vi "NPL Joerger Dust Ablation.vi"() -> ()   [LabVIEW 2013]
uses:
  <vilib>/Utility/file.llb/Write To Spreadsheet File (DBL).vi
panel:
  out "Event Num":i32
  out "Waveforms":ext[][](graph)
  out "Waveform 17-32":ext[][](graph)
  out "State":i32
  in  "Save Files":bool
  out "Waveform output":ext[][](array[numeric])
  out "8bit integer 3":i8 format="%08b"
  out "8bit integer 2":i8 format="%08b"
  out "8bit integer":i8 format="%08b"
  out "dt":dbl
  in  "Change folder":bool
  out "Waveform Folder":path
  in  "Manual Arm":bool
  out "Waveform 1-16":ext[][](graph)
  out "# Channels Plotted":i32
  in  "How Many Cards?":u16(ring) items=["2", "3"]
  out "Electrons Min Signal":cluster{i32[], "Ions Max Value":ext[]}(graph)
  out "Ions Max Signal":cluster{i32[], "Ions Max Value":ext[]}(graph)
  out "Sec. Since Last Read":dbl
  in  "stop":bool
  in  "Arm":bool
  in  "Number of Channels":u8=16
  in  "# Samples":u32=2000 min=1 max=262143 step=1
  out "Length of Sample":dbl caption="s" format="%^#_3g"
  in  "Acquisition Rate 2":u16(ring)=2 items=["40 MHz", "20 MHz", "10 MHz", "5 MHz", "2.5 MHz", "1 MHz", "100 kHz", "10 kHz"]
  # "0"
  # "1"
  # "Sampling Controls"
  # "Sampling Info"
  # "Triggering Setup"
  # "2"
  # "3"
  # "4"
  # "5"
  # "6"
  # "7"
  # "8"
  # "9"
  # "10"
  # "11"
  # "This resets the\nwaveform count \nto zero when saving\nwaveforms"
  # "12"
  # "13"
  # "14"
  # "15"
  # "0"
  # "1"
  # "2"
  # "3"
  # "4"
  # "5"
  # "6"
  # "7"
  # "8"
  # "9"
  # "10"
  # "11"
  # "12"
  # "13"
  # "14"
  # "15"
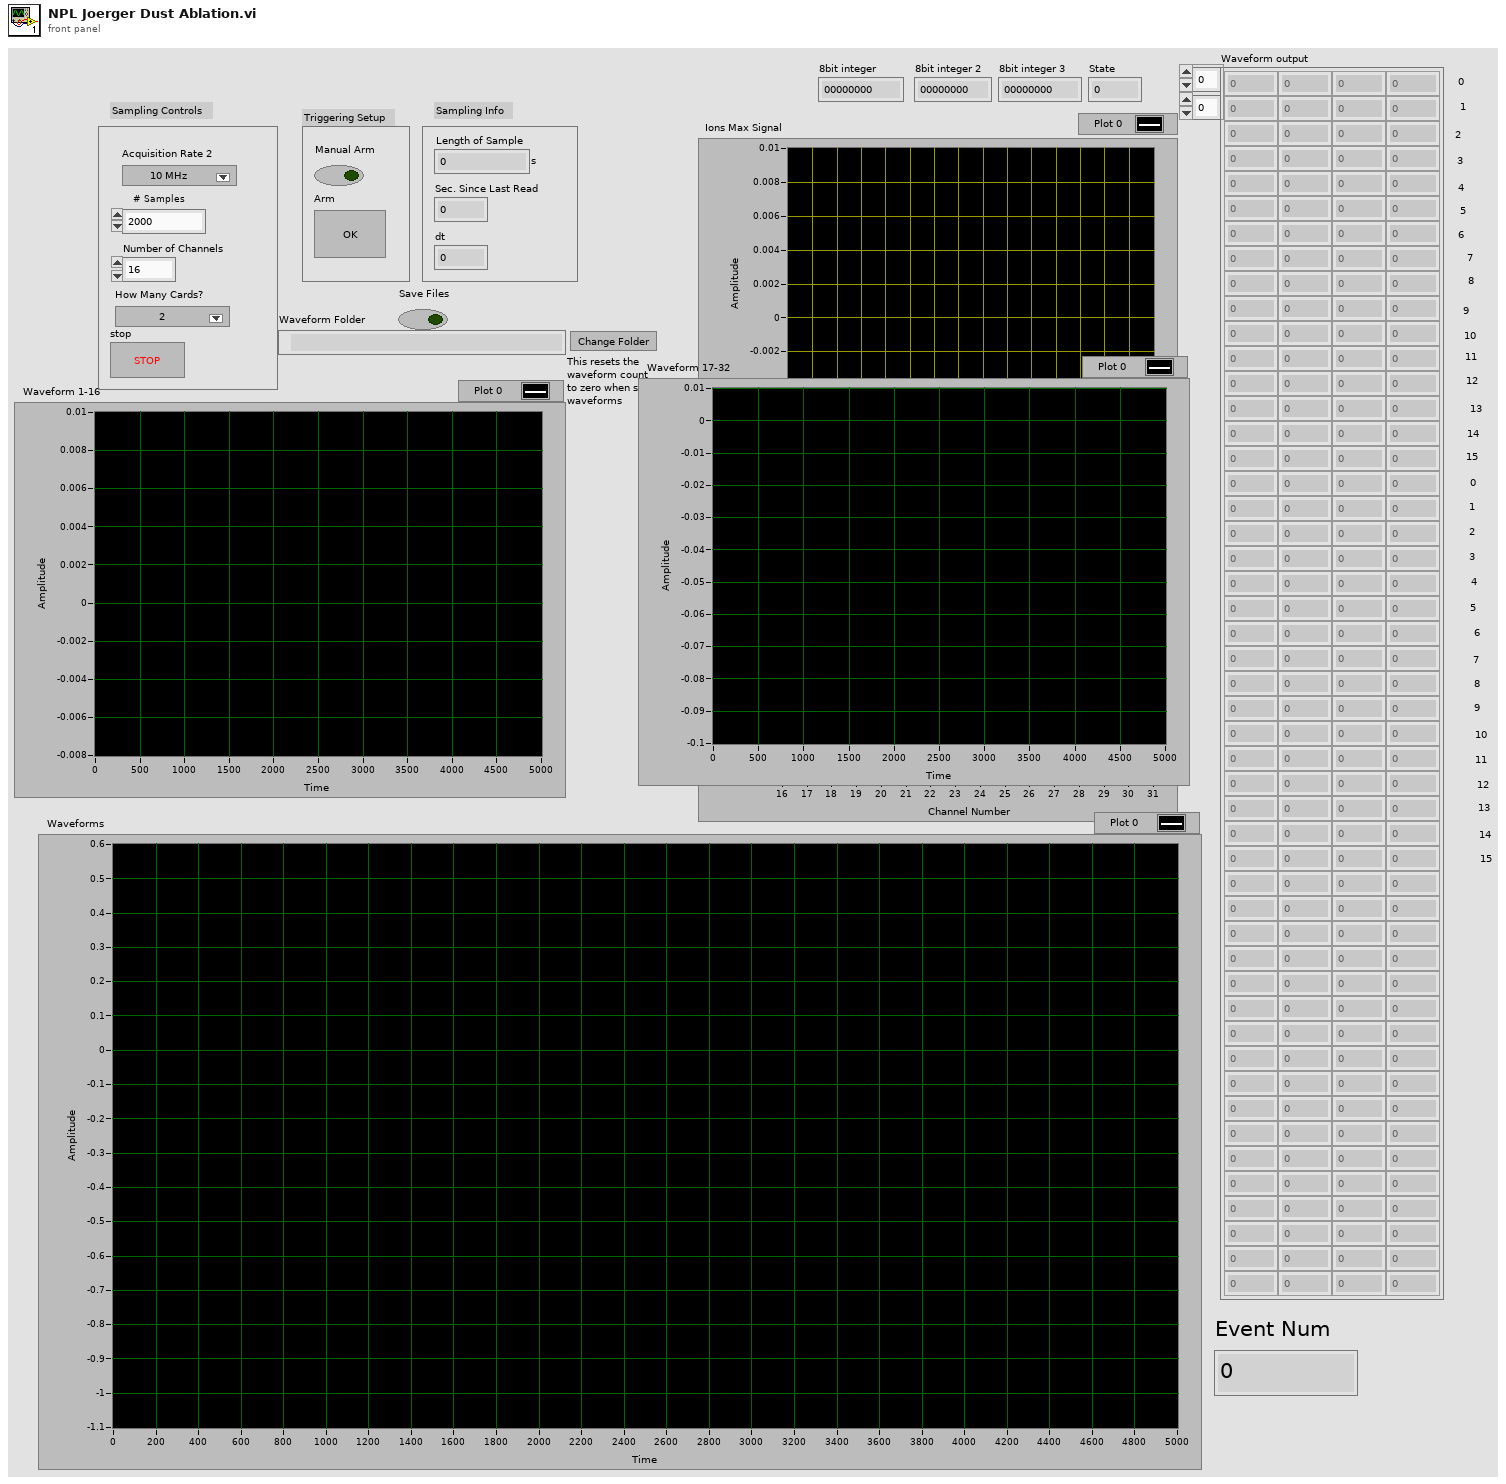
[diagram p1: front panel]
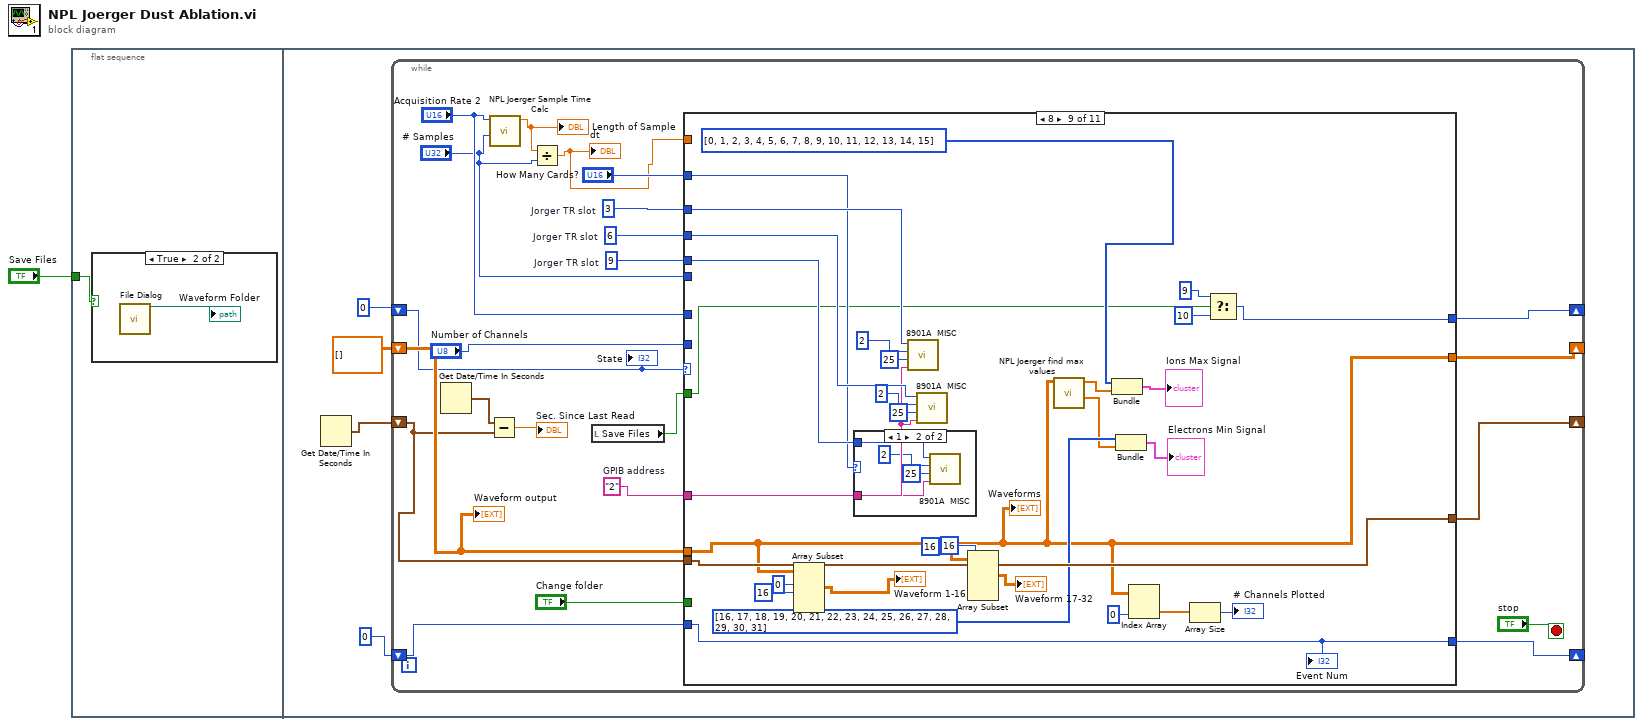
[diagram p0: block diagram]
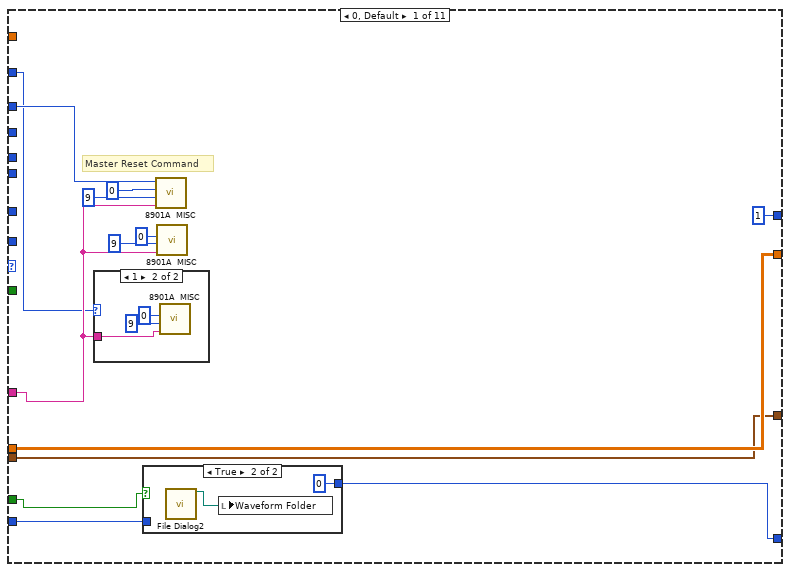
[diagram p3: hidden frame]
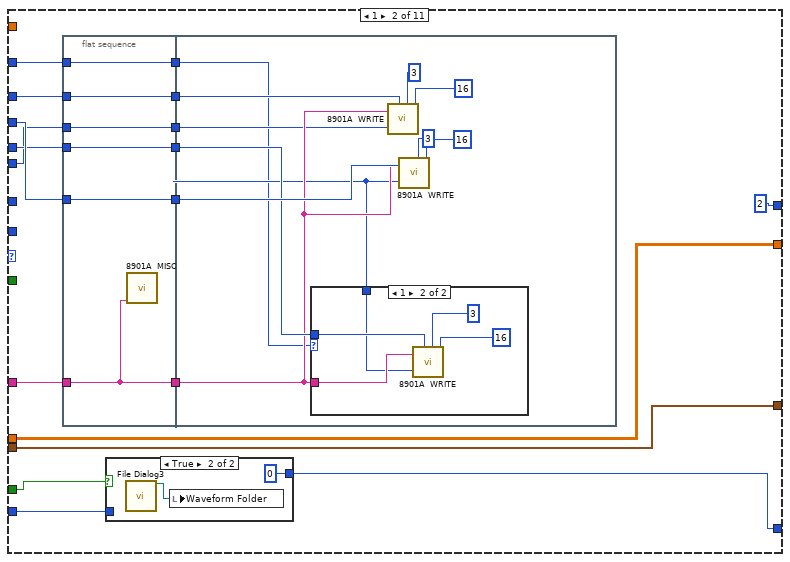
[diagram p6: hidden frame]
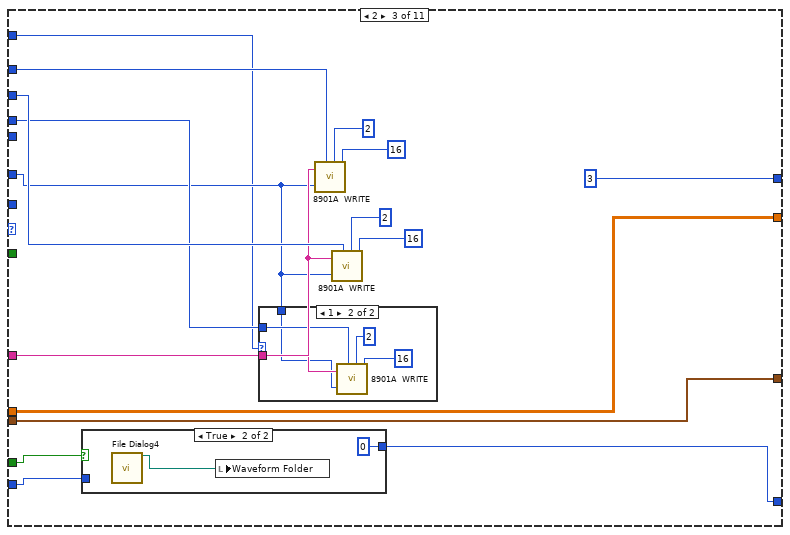
[diagram p9: hidden frame]
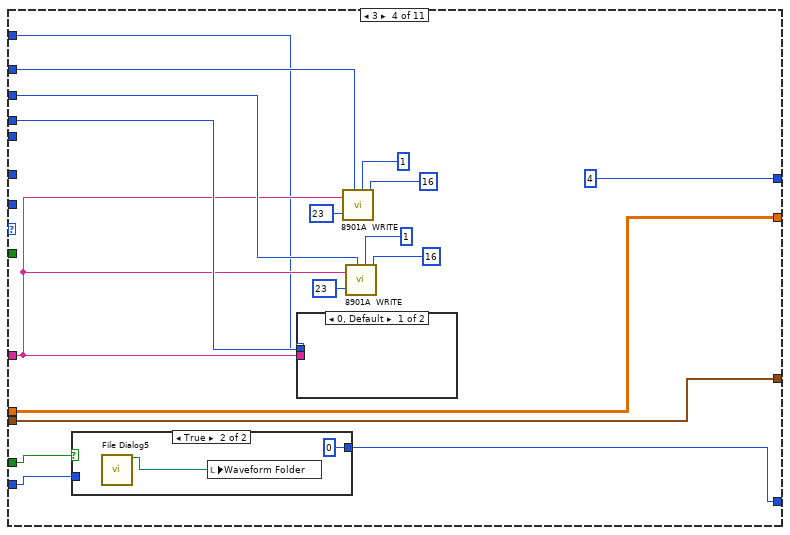
[diagram p12: hidden frame]
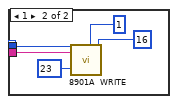
[diagram p14: hidden frame]
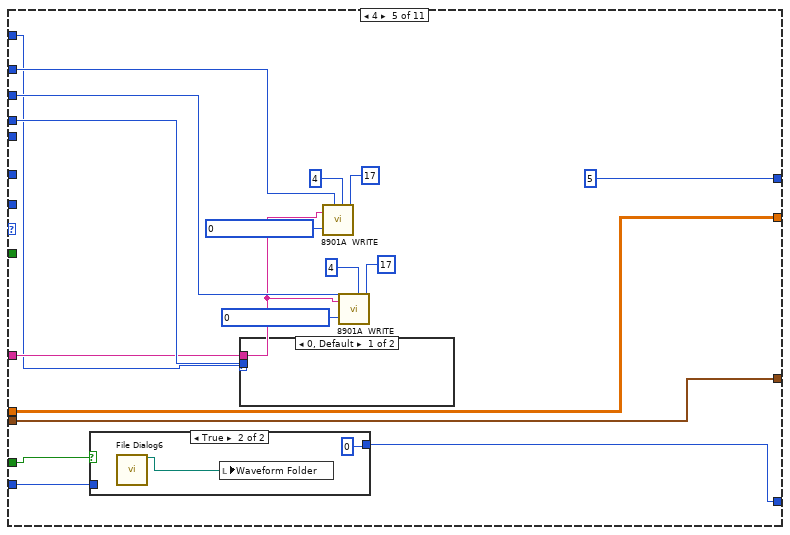
[diagram p15: hidden frame]
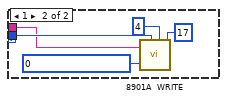
[diagram p17: hidden frame]
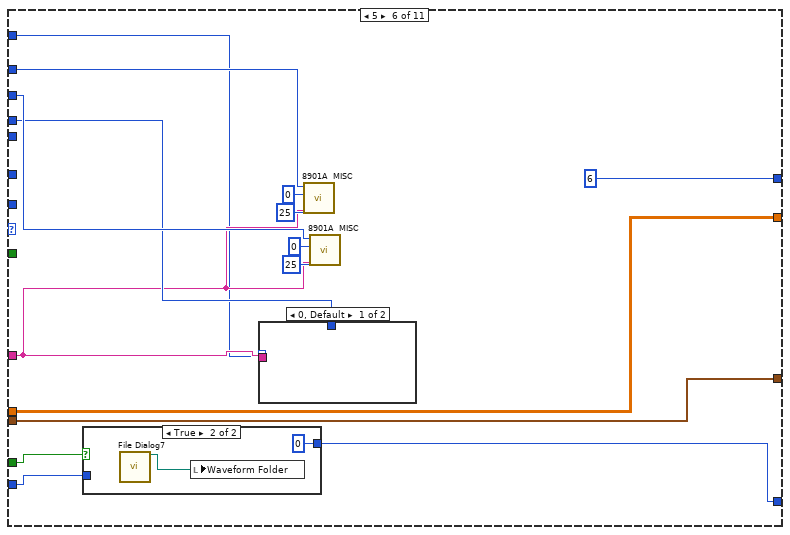
[diagram p18: hidden frame]
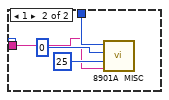
[diagram p20: hidden frame]
diagram:
  n1 = flat-sequence {
    tunnel: "Save Files" -> [w2]
    frame #0 {
      n2 = case shown="True" w2 {
        frame False {
        }
        frame True {
          n3 = call "File Dialog"() -> ("selected path"=→"Waveform Folder":path)  [unwired: 12 in, 3 out]
        }
      }
    }
    frame #1 {
      n4 = Get Date/Time In Seconds() -> (seconds since 1Jan1904=w5:timestamp)
      n5 = while {
        shift-right: [w28] -> _
        shift-left: 0 -> [w23]
        shift-right: [w25] -> _
        shift-left: ext[][] [] ("output") -> [w24]
        shift-right: [w22] -> _
        shift-left: w5 -> [w20]
        shift-right: [w12] -> _
        shift-left: 0 -> [w13]
        stop <- "stop" stop-if-true
        w17 = u8 9  # Jorger TR slot
        w18 = u8 6  # Jorger TR slot
        w30 = u8 3  # Jorger TR slot
        w29 = "2"  # GPIB address
        n6 = Get Date/Time In Seconds() -> (seconds since 1Jan1904=w21:timestamp)
        n7 = Subtract(x=w21, y=w20) -> (x-y=→"Sec. Since Last Read":dbl)
        n8 = call "NPL Joerger Sample Time Calc.vi"("# Samples"="# Samples", "Acquisition Rate"="Acquisition Rate 2") -> ("Sample Time"=w11:dbl)  [unwired: 9 in]
        "Length of Sample" <- w11
        n9 = Divide(x=w11, y="# Samples") -> (x/y=w9:dbl)
        "dt" <- w9
        n10 = local read "Save Files"() -> (w8:bool)
        n11 = case shown="8" w23 {
          tunnel: w30 -> [w37 w67 w107 w132 w157 w180 w226 w262 w355 _ _]
          tunnel: w29 -> [w38 w61 w97 w120 w145 w170 w197 w263 w347 _ _]
          tunnel: [1 ("f") 2 3 4 5 6 w199 8 ("f") w332 10 ("f") w387] -> w28
          tunnel: "# Samples" -> [_ w60 _ _ _ _ _ w259 _ _ _]
          tunnel: "Acquisition Rate 2" -> [_ _ w96 _ _ _ _ _ _ _ _]
          tunnel: "Number of Channels" -> [_ _ _ _ _ _ _ w260 _ _ _]
          tunnel: [w43 w65 w103 w127 w152 w176 w212 w248 w325 w378 w386] -> w25
          tunnel: w24 -> [w43 w65 w103 w127 w152 w176 w212 _ w325 w378 w386]
          tunnel: w20 -> [w42 w64 w102 w126 w151 w175 w211 _ w352 w366 w389]
          tunnel: [w42 w64 w102 w126 w151 w175 w211 w258 w352 w366 w389] -> w22
          tunnel: w18 -> [_ w63 w99 w122 w147 w172 w208 w256 w349 _ _]
          tunnel: w17 -> [_ w62 w98 w121 w146 w171 w198 w255 w348 _ _]
          tunnel: "How Many Cards?" -> [w31 w59 w95 w119 w144 w169 w191 w247 w340 _ _]
          tunnel: "Change folder" -> [w41 w58 w94 w118 w143 w168 w190 _ _ _ _]
          tunnel: w13 -> [w39 w56 w92 w116 w141 w166 w188 w246 w336 w369 w385]
          tunnel: [w40 w57 w93 w117 w142 w167 w189 w245 w336 w369 w385] -> w12
          tunnel: w9 -> [_ _ _ _ _ _ _ _ _ w368 _]
          tunnel: w8 -> [_ _ _ _ _ _ _ _ w335 _ _]
          frame 0, Default {
            # "Master Reset Command"
            n12 = case shown="1" w31 {
              tunnel: w38 -> [_ w46]
              frame 0, Default {
              }
              frame 1 {
                n13 = call <instrlib>:"8901A  MISC.vi"("GPIB address"=w46, "f"=u8 9, "a"=u8 0) -> ()  [unwired: 1 in]
              }
            }
            n14 = case shown="True" w41 {
              tunnel: [w47 0] -> w40
              tunnel: w39 -> [w47 _]
              frame False {
              }
              frame True {
                n15 = call "File Dialog2"() -> ("selected path"=w49:path)  [unwired: 12 in, 3 out]
                n16 = local write "Waveform Folder"(w49) -> ()
              }
            }
            n17 = call <instrlib>:"8901A  MISC.vi"("GPIB address"=w38, "f"=u8 9, "a"=u8 0, "n"=w37) -> ()
            n18 = call <instrlib>:"8901A  MISC.vi"("GPIB address"=w38, "f"=u8 9, "a"=u8 0) -> ()  [unwired: 1 in]
          }
          frame 1 {
            n19 = flat-sequence {
              tunnel: w59 -> [w69]
              tunnel: w60 -> [w70]
              tunnel: w61 -> [w68]
              tunnel: w62 -> [w71]
              tunnel: w63 -> [w72]
              tunnel: w67 -> [w73]
              tunnel: [w73] -> w55
              tunnel: [w72] -> w54
              tunnel: [w71] -> w53
              tunnel: [w68] -> w52
              tunnel: [w70] -> w51
              tunnel: [w69] -> w50
              tunnel: w55 -> [w83]
              tunnel: w54 -> [w78]
              tunnel: w53 -> [w77]
              tunnel: w52 -> [w76]
              tunnel: w51 -> [w75]
              tunnel: w50 -> [w74]
              frame #0 {
                n20 = call <instrlib>:"8901A  MISC.vi"("GPIB address"=w68) -> ()  [unwired: 3 in]
              }
              frame #1 {
                n21 = case shown="1" w74 {
                  tunnel: w77 -> [_ w86]
                  tunnel: w76 -> [_ w85]
                  tunnel: w75 -> [_ w84]
                  frame 0, Default {
                  }
                  frame 1 {
                    n22 = call <instrlib>:"8901A  WRITE.vi"("data"=w84, "GPIB address"=w85, "n"=w86, "a"=u8 3, "f"=u8 16) -> ()  [unwired: 1 in]
                  }
                }
                n23 = call <instrlib>:"8901A  WRITE.vi"("data"=w75, "GPIB address"=w76, "n"=w83, "a"=u8 3, "f"=u8 16) -> ()  [unwired: 1 in]
                n24 = call <instrlib>:"8901A  WRITE.vi"("data"=w75, "GPIB address"=w76, "n"=w78, "a"=u8 3, "f"=u8 16) -> ()  [unwired: 1 in]
              }
            }
            n25 = case shown="True" w58 {
              tunnel: [w89 0] -> w57
              tunnel: w56 -> [w89 _]
              frame False {
              }
              frame True {
                n26 = call "File Dialog3"() -> ("selected path"=w91:path)  [unwired: 12 in, 3 out]
                n27 = local write "Waveform Folder"(w91) -> ()
              }
            }
          }
          frame 2 {
            n28 = case shown="True" w94 {
              tunnel: [w108 0] -> w93
              tunnel: w92 -> [w108 _]
              frame False {
              }
              frame True {
                n29 = call "File Dialog4"() -> ("selected path"=w110:path)  [unwired: 12 in, 3 out]
                n30 = local write "Waveform Folder"(w110) -> ()
              }
            }
            n31 = case shown="1" w95 {
              tunnel: w98 -> [_ w113]
              tunnel: w97 -> [_ w112]
              tunnel: w96 -> [_ w111]
              frame 0, Default {
              }
              frame 1 {
                n32 = call <instrlib>:"8901A  WRITE.vi"("data"=w111, "GPIB address"=w112, "n"=w113, "a"=u8 2, "f"=u8 16) -> ()  [unwired: 1 in]
              }
            }
            n33 = call <instrlib>:"8901A  WRITE.vi"("data"=w96, "GPIB address"=w97, "n"=w107, "a"=u8 2, "f"=u8 16) -> ()  [unwired: 1 in]
            n34 = call <instrlib>:"8901A  WRITE.vi"("data"=w96, "GPIB address"=w97, "n"=w99, "a"=u8 2, "f"=u8 16) -> ()  [unwired: 1 in]
          }
          frame 3 {
            n35 = case shown="True" w118 {
              tunnel: [w133 0] -> w117
              tunnel: w116 -> [w133 _]
              frame False {
              }
              frame True {
                n36 = call "File Dialog5"() -> ("selected path"=w135:path)  [unwired: 12 in, 3 out]
                n37 = local write "Waveform Folder"(w135) -> ()
              }
            }
            n38 = case shown="0, Default" w119 {
              tunnel: w121 -> [_ w137]
              tunnel: w120 -> [_ w136]
              frame 0, Default {
              }
              frame 1 {
                n39 = call <instrlib>:"8901A  WRITE.vi"("data"=23, "GPIB address"=w136, "n"=w137, "a"=u8 1, "f"=u8 16) -> ()  [unwired: 1 in]
              }
            }
            n40 = call <instrlib>:"8901A  WRITE.vi"("data"=23, "GPIB address"=w120, "n"=w132, "a"=u8 1, "f"=u8 16) -> ()  [unwired: 1 in]
            n41 = call <instrlib>:"8901A  WRITE.vi"("data"=23, "GPIB address"=w120, "n"=w122, "a"=u8 1, "f"=u8 16) -> ()  [unwired: 1 in]
          }
          frame 4 {
            n42 = case shown="True" w143 {
              tunnel: [w158 0] -> w142
              tunnel: w141 -> [w158 _]
              frame False {
              }
              frame True {
                n43 = call "File Dialog6"() -> ("selected path"=w160:path)  [unwired: 12 in, 3 out]
                n44 = local write "Waveform Folder"(w160) -> ()
              }
            }
            n45 = case shown="0, Default" w144 {
              tunnel: w146 -> [_ w162]
              tunnel: w145 -> [_ w161]
              frame 0, Default {
              }
              frame 1 {
                n46 = call <instrlib>:"8901A  WRITE.vi"("data"=0, "GPIB address"=w161, "n"=w162, "a"=u8 4, "f"=u8 17) -> ()  [unwired: 1 in]
              }
            }
            n47 = call <instrlib>:"8901A  WRITE.vi"("data"=0, "GPIB address"=w145, "n"=w157, "a"=u8 4, "f"=u8 17) -> ()  [unwired: 1 in]
            n48 = call <instrlib>:"8901A  WRITE.vi"("data"=0, "GPIB address"=w145, "n"=w147, "a"=u8 4, "f"=u8 17) -> ()  [unwired: 1 in]
          }
          frame 5 {
            n49 = case shown="True" w168 {
              tunnel: [w181 0] -> w167
              tunnel: w166 -> [w181 _]
              frame False {
              }
              frame True {
                n50 = call "File Dialog7"() -> ("selected path"=w183:path)  [unwired: 12 in, 3 out]
                n51 = local write "Waveform Folder"(w183) -> ()
              }
            }
            n52 = case shown="0, Default" w169 {
              tunnel: w171 -> [_ w185]
              tunnel: w170 -> [_ w184]
              frame 0, Default {
              }
              frame 1 {
                n53 = call <instrlib>:"8901A  MISC.vi"("GPIB address"=w184, "f"=u8 25, "a"=u8 0, "n"=w185) -> ()
              }
            }
            n54 = call <instrlib>:"8901A  MISC.vi"("GPIB address"=w170, "f"=u8 25, "a"=u8 0, "n"=w180) -> ()
            n55 = call <instrlib>:"8901A  MISC.vi"("GPIB address"=w170, "f"=u8 25, "a"=u8 0, "n"=w172) -> ()
          }
          frame 6 {
            # "Check status register to see that\nmodule is neither armed nor active\n(bits R1 & R2 = 0)."
            n56 = case shown="True" w190 {
              tunnel: [w227 0] -> w189
              tunnel: w188 -> [w227 _]
              frame False {
              }
              frame True {
                n57 = call "File Dialog8"() -> ("selected path"=w229:path)  [unwired: 12 in, 3 out]
                n58 = local write "Waveform Folder"(w229) -> ()
              }
            }
            n59 = case shown="1" w191 {
              tunnel: w198 -> [_ w242]
              tunnel: w197 -> [_ w241]
              tunnel: [FALSE w231] -> w193
              frame 0, Default {
              }
              frame 1 {
                n60 = call <instrlib>:"8901A READ 8.vi"("GPIB address"=w241, "n"=w242, "a"=u8 0, "f"=u8 1) -> ("output"=w232:ext)  [unwired: 3 in]
                n61 = To Byte Integer(number=w232) -> (8bit integer=w240:i8)
                "8bit integer 3" <- w240
                n62 = And(x=w240, y=i8 3) -> (x .and. y?=w238:i8)
                n63 = Number To Boolean Array(number=w238) -> (Boolean array=w236:bool[])
                n64 = Index Array(array=w236, index=0) -> (element=w233:bool)
                n65 = Index Array(array=w236, index=1) -> (element=w234:bool)
                n66 = Or(x=w233, y=w234) -> (x .or. y?=w231:bool)
              }
            }
            n67 = call <instrlib>:"8901A READ 8.vi"("GPIB address"=w197, "n"=w226, "a"=u8 0, "f"=u8 1) -> ("output"=w223:ext)  [unwired: 3 in]
            n68 = call <instrlib>:"8901A READ 8.vi"("GPIB address"=w197, "n"=w208, "a"=u8 0, "f"=u8 1) -> ("output"=w196:ext)  [unwired: 3 in]
            n69 = To Byte Integer(number=w223) -> (8bit integer=w222:i8)
            "8bit integer" <- w222
            n70 = To Byte Integer(number=w196) -> (8bit integer=w200:i8)
            "8bit integer 2" <- w200
            n71 = And(x=w222, y=i8 3) -> (x .and. y?=w220:i8)
            n72 = And(x=w200, y=i8 3) -> (x .and. y?=w202:i8)
            n73 = Number To Boolean Array(number=w220) -> (Boolean array=w218:bool[])
            n74 = Number To Boolean Array(number=w202) -> (Boolean array=w204:bool[])
            n75 = Index Array(array=w218, index=0) -> (element=w215:bool)
            n76 = Index Array(array=w218, index=1) -> (element=w216:bool)
            n77 = Index Array(array=w204, index=0) -> (element=w207:bool)
            n78 = Index Array(array=w204, index=1) -> (element=w206:bool)
            n79 = Or(x=w215, y=w216) -> (x .or. y?=w195:bool)
            n80 = Or(x=w207, y=w206) -> (x .or. y?=w194:bool)
            n81 = Compound Arithmetic op=OR(w195, w194, w193) -> (w192:bool)
            n82 = Select(t=6, s=w192, f=7) -> (s? t:f=w199:i32)
          }
          frame 7 {
            # "Increment\nWaveform #"
            # "0...15 card 1\n16...31 card 2\n32...47 card 3"
            # "Read out the data from the number of channels\nspecified."
            n83 = Increment(x=w246) -> (x+1=w245:i32)
            n84 = for {
              N: w260 -> [_]
              tunnel: w263 -> [w273]
              tunnel: w262 -> [w283]
              tunnel: w259 -> [w271]
              tunnel: [w280] -> w257 mode=indexing
              tunnel: w256 -> [w277]
              tunnel: [w276] -> w254 mode=indexing
              tunnel: [w275] -> w253 mode=indexing
              tunnel: w255 -> [w274]
              tunnel: w247 -> [w270]
              i -> [w272]
              n85 = case shown="1" w270 {
                tunnel: [ext[] [] ("output") w289] -> w275
                tunnel: w274 -> [_ w288]
                tunnel: w273 -> [_ w287]
                tunnel: w272 -> [_ w286]
                tunnel: w271 -> [_ w285]
                frame 0, Default {
                }
                frame 1 {
                  n86 = flat-sequence {
                    tunnel: w287 -> [w293]
                    tunnel: w288 -> [w292]
                    tunnel: [w293] -> w291
                    tunnel: [w292] -> w290
                    tunnel: w291 -> [w302]
                    tunnel: w290 -> [w301]
                    tunnel: w286 -> [w299]
                    tunnel: [w297] -> _
                    tunnel: [w298] -> w289
                    tunnel: w285 -> [w297]
                    frame #0 {
                      n87 = call <instrlib>:"8901A  WRITE.vi"("data"=0, "GPIB address"=w293, "n"=w292, "a"=u8 1, "f"=u8 17) -> ()  [unwired: 1 in]
                    }
                    frame #1 {
                      n88 = call <instrlib>:"8901A BLOCK READ 24.vi"("f"=u8 2, "a"=w299, "n"=w301, "GPIB address"=w302, "# points to read"=w297) -> ("output"=w298:ext[])  [unwired: 4 in]
                    }
                  }
                }
              }
              n89 = flat-sequence {
                tunnel: w273 -> [w315]
                tunnel: w283 -> [w314]
                tunnel: [w315] -> w282
                tunnel: [w314] -> w281
                tunnel: w282 -> [w324]
                tunnel: w281 -> [w323]
                tunnel: w272 -> [w321]
                tunnel: w271 -> [w320]
                tunnel: [w319] -> w280
                frame #0 {
                  n90 = call <instrlib>:"8901A  WRITE.vi"("data"=0, "GPIB address"=w315, "n"=w314, "a"=u8 1, "f"=u8 17) -> ()  [unwired: 1 in]
                }
                frame #1 {
                  n91 = call <instrlib>:"8901A BLOCK READ 24.vi"("f"=u8 2, "a"=w321, "n"=w323, "GPIB address"=w324, "# points to read"=w320) -> ("output"=w319:ext[])  [unwired: 4 in]
                }
              }
              n92 = flat-sequence {
                tunnel: w273 -> [w304]
                tunnel: w277 -> [w303]
                tunnel: [w304] -> w279
                tunnel: [w303] -> w278
                tunnel: w279 -> [w313]
                tunnel: w278 -> [w312]
                tunnel: w272 -> [w310]
                tunnel: w271 -> [w309]
                tunnel: [w308] -> w276
                frame #0 {
                  n93 = call <instrlib>:"8901A  WRITE.vi"("data"=0, "GPIB address"=w304, "n"=w303, "a"=u8 1, "f"=u8 17) -> ()  [unwired: 1 in]
                }
                frame #1 {
                  n94 = call <instrlib>:"8901A BLOCK READ 24.vi"("f"=u8 2, "a"=w310, "n"=w312, "GPIB address"=w313, "# points to read"=w309) -> ("output"=w308:ext[])  [unwired: 4 in]
                }
              }
            }
            n95 = call "NPL Joerger ADC Convert.vi"("Input"=w257) -> ("Output"=w252:ext[][])  [unwired: 10 in]
            n96 = call "NPL Joerger ADC Convert.vi"("Input"=w254) -> ("Output"=w250:ext[][])  [unwired: 10 in]
            n97 = Insert Into Array(array=w252, index (row)=16, new element=w250) -> (w249:ext[][])  [unwired: 1 in]
            n98 = case shown="1" w247 {
              tunnel: w253 -> [_ w269]
              tunnel: w249 -> [w264 w268]
              tunnel: [w264 w265] -> w248
              frame 0, Default {
              }
              frame 1 {
                n99 = call "NPL Joerger ADC Convert.vi"("Input"=w269) -> ("Output"=w266:ext[][])  [unwired: 10 in]
                n100 = Insert Into Array(array=w268, index (row)=32, new element=w266) -> (w265:ext[][])  [unwired: 1 in]
              }
            }
            n101 = Get Date/Time In Seconds() -> (seconds since 1Jan1904=w258:timestamp)
          }
          frame 8 {
            n102 = Array Subset(array=w325, index (row)=0 ("index"), length (row)=16 ("length")) -> (→"Waveform 1-16":ext[][])  [unwired: 2 in]
            n103 = case shown="1" w340 {
              tunnel: w348 -> [_ w357]
              tunnel: w347 -> [_ w356]
              frame 0, Default {
              }
              frame 1 {
                n104 = call <instrlib>:"8901A  MISC.vi"("GPIB address"=w356, "f"=u8 25, "a"=u8 2, "n"=w357) -> ()
              }
            }
            n105 = call <instrlib>:"8901A  MISC.vi"("GPIB address"=w347, "f"=u8 25, "a"=u8 2, "n"=w355) -> ()
            n106 = call <instrlib>:"8901A  MISC.vi"("GPIB address"=w347, "f"=u8 25, "a"=u8 2, "n"=w349) -> ()
            n107 = Array Subset(array=w325, index (row)=16 ("index"), length (row)=16 ("length")) -> (→"Waveform 17-32":ext[][])  [unwired: 2 in]
            n108 = call "NPL Joerger find max values.vi"("Input"=w325) -> ("Electrons Min Value"=w342:ext[], "Ions Max Value"=w345:ext[])  [unwired: 9 in]
            n109 = Bundle(i32[] [0, 1, 2, 3, 4, 5, 6, 7, 8, 9, 10, 11, 12, 13, 14, 15], "Ions Max Value"=w345) -> (→"Ions Max Signal":cluster{i32[], "Ions Max Value":ext[]})  [unwired: 1 in]
            n110 = Bundle(i32[] [16, 17, 18, 19, 20, 21, 22, 23, 24, 25, 26, 27, 28, 29, 30, 31], "Electrons Min Value"=w342) -> (→"Electrons Min Signal":cluster{i32[], "Electrons Min Value":ext[]})  [unwired: 1 in]
            n111 = Index Array(array=w325, index (col)=0 ("disabled index (col)")) -> (element=w338:ext[])  [unwired: 1 in]
            n112 = Array Size(array=w338) -> (size(s)=→"# Channels Plotted":i32)
            n113 = Select(t=9 ("f"), s=w335, f=10) -> (s? t:f=w332:i32)
            "Waveforms" <- w325
            "Event Num" <- w336
          }
          frame 9 {
            # "Number of Waveforms"
            n114 = local read "Waveform Folder"() -> (w375:path)
            n115 = Index Array(array=w378, index (col)=0 ("disabled index (col)")) -> (element=w381:ext[])  [unwired: 1 in]
            n116 = Number To Decimal String(number=w369) -> (decimal integer string=w364:string)  [unwired: 1 in]
            n117 = Path To String(path=w375) -> (string=w374:string)
            n118 = Array Size(array=w381) -> (size(s)=w377:i32)
            n119 = call "timestamp_conversion.vi"("Time Stamp"=w366) -> ("Integer Time"=w362:i64)  [unwired: 8 in, 1 out]
            n120 = Number To Decimal String(number=w362) -> (decimal integer string=w361:string)  [unwired: 1 in]
            n121 = for {
              N: w377 -> [_]
              tunnel: w368 -> [w384]
              tunnel: [w382] -> w376 mode=indexing
              i -> [w383]
              n122 = Multiply(x=w384, y=w383) -> (x*y=w382:dbl)
            }
            n123 = Concatenate Strings(w374, "\\AblationEvent", w364, "_" ("string"), w361, ".csv" ("string")) -> (w373:string)
            n124 = String To Path(string=w373) -> (path=w372:path)
            n125 = Insert Into Array(array=w378, index (row)=w377, new element=w376) -> (w367:ext[][])  [unwired: 1 in]
            n126 = call-poly <vilib>:"Write To Spreadsheet File.vi"("delimiter (\\t)"="," ("delimiter (\\t)"), "format (%.3f)"="%.10f", "2D data"=w367, "file path (dialog if empty)"=w372) -> ()  [unwired: 4 in, 1 out]
          }
          frame 10 {
            n127 = case shown="True" "Manual Arm" {
              tunnel: [1 ("f") w391] -> w387
              frame False {
              }
              frame True {
                n128 = Select(t=1, s="Arm", f=10) -> (s? t:f=w391:i32)
              }
            }
          }
        }
        "Waveform output" <- w24
        "State" <- w23
      }
    }
  }
